vi "Read PAE Pins.vi"(8 "error in (no error)":errorcluster, 11 "Power Sweep in":refnum<class "Power Sweep.lvclass">) -> (0 "error out":errorcluster, 2 "PAE Pins":string[](array[string]), 3 "Power Sweep out":refnum<class "Power Sweep.lvclass">)   [LabVIEW 2018, in "Power Sweep.lvlib" / "Power Sweep.lvclass"]
uses:
  Power Sweep.lvclass
  Power Sweep.lvclass/Power Sweep.ctl
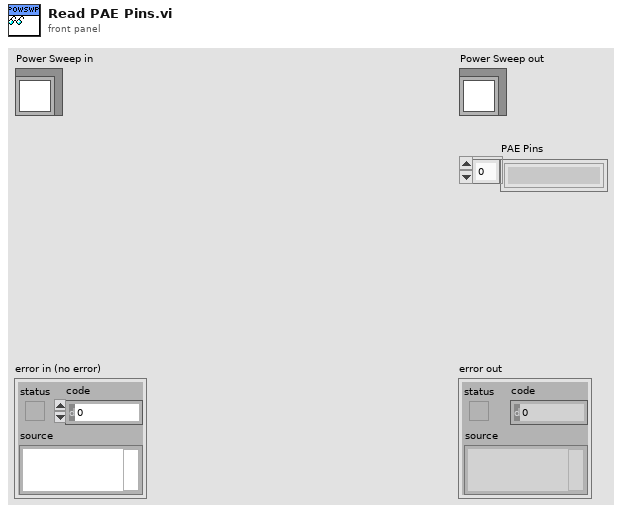
[diagram p1: front panel]
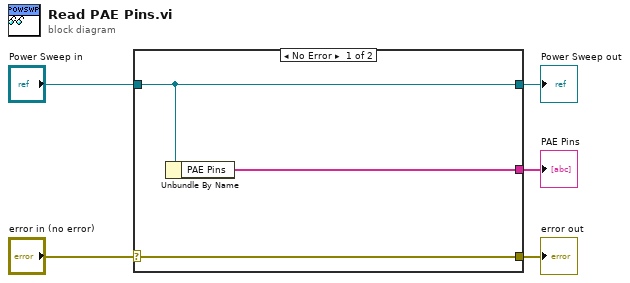
[diagram p0: block diagram]
diagram:
  n1 = case shown="No Error" "error in (no error)" {
    selector: "error in (no error)" -> [w8 w9]
    tunnel: [w8 w9] -> w4
    tunnel: [w7 w10] -> w2
    tunnel: "Power Sweep in" -> [w7 w10]
    tunnel: [w6 _] -> w1
    frame No Error {
      n2 = Unbundle By Name(w7) -> ("PAE Pins"=w6:string[])
    }
    frame Error {
    }
  }
  "error out" <- w4
  "Power Sweep out" <- w2
  "PAE Pins" <- w1
